vi "ReadChanValue.vi"(8 "error in (no error)":errorcluster, 10 "nScale":i32, 11 "nWhichChan":i32) -> (0 "error out":errorcluster, 1 "*pnChanSpanOffset":i32, 2 "*pnChanZeroOffset":i32, 3 "Return Code":i32, 5 "*pnChanValue":i32)   [LabVIEW 2015]
doc: "Call this to initiate a connection with the UUT. \nDetail: \nint ConnectToOthello (aMEScope_ReadChanVal\nDescription:\nThis function will read an analog channel ADC offset. Calibration values are also returned to properly calculate the final result.\nDetail:\nint MEScope_ReadChanVal (\nint nWhichChan, \nint nScale, \nint *pnChanValue, \nint *pnChanZeroOffset,\nint *pnChanSpanOffset\n);\nParameters:\nint nWhichChan - which channel to use (CHANNEL_1 or CHANNEL_2)\n\nint nScale - which scale to use (CHANNEL_SCALE_1V to CHANNEL_SCALE_400V)\n\nint *pnChanValue - pointer to an integer, filled with the ADC count value for the channel, scale and input requested.\n\nint * pnChanZeroOffset - pointer to an integer, filled with the zero offset calibration value for the requested channel, scale and input. It can be NULL if the data isn't required.\n\nint * pnChanSpanOffset - pointer to an integer, filled with the span offset calibration value for the requested channel, scale and input. It can be NULL if the data isn't required.\n\nReturn Values:\nThis function returns a 0 if the function completed successfully. A non-zero return code will indicate error. \nRemarks:\nChannel definitions:\n#define CHANNEL_1 0\n#define CHANNEL_2 1\n\nScale definitions:\n#define CHANNEL_SCALE_1V 0\n#define CHANNEL_SCALE_2V 1\n#define CHANNEL_SCALE_5V 2\n#define CHANNEL_SCALE_10V 3\n#define CHANNEL_SCALE_20V 4\n#define CHANNEL_SCALE_50V 5\n#define CHANNEL_SCALE_100V 6\n#define CHANNEL_SCALE_200V 7\n#define CHANNEL_SCALE_400V 8\n\nSee Appendix 4 for details on converting ADC reading into a measurement.\nSerial Command packet: \nn/a\n\nint nPort\n);\n \nParameters:\nint nPort - Port used by USB serial device\nReturn Values:\nA returned value of 0 indicates success. A non-zero return code will indicate error.\nRemarks:"
uses:
  ScannerDiagDLL.dll
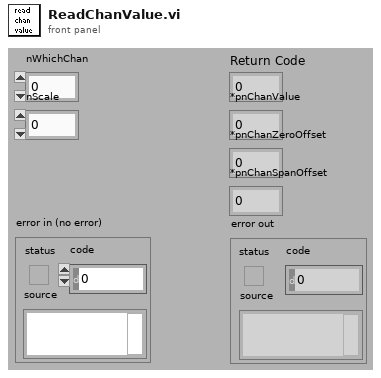
[diagram p1: front panel]
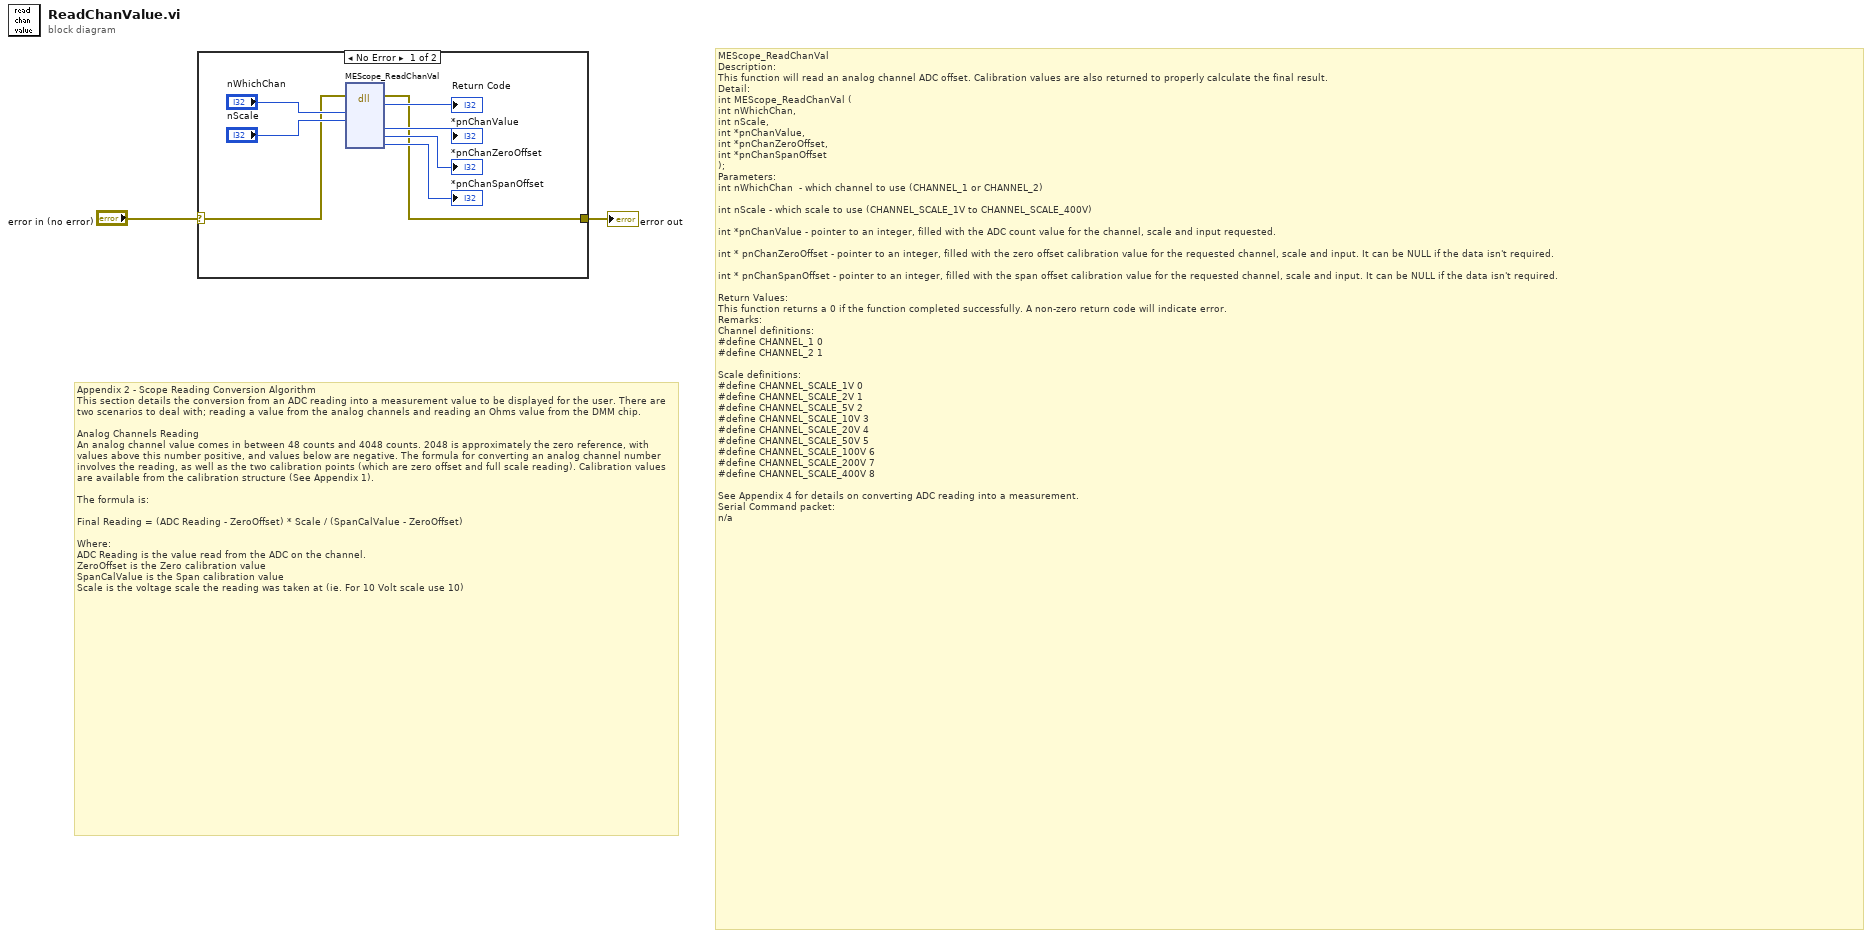
[diagram p0: block diagram]
diagram:
  # "Appendix 2 - Scope Reading Conversion Algorithm\nThis section details the conversion from an ADC reading into a measurement value to be displayed for the user. There are two scenarios to deal with; reading a value from the analog channels and reading an Ohms value from the DMM chip.\n\nAnalog Channels Reading\nAn analog channel value comes in between 48 counts and 4048 counts. 2048 is approximately the zero reference, with values above this number positive, and values below are negative. The formula for converting an analog channel number involves the reading, as well as the two calibration points (which are zero offset and full scale reading). Calibration values are available from the calibration structure (See Appendix 1). \n\nThe formula is:\n\nFinal Reading = (ADC Reading - ZeroOffset) * Scale / (SpanCalValue - ZeroOffset)\n\nWhere:\nADC Reading is the value read from the ADC on the channel.\nZeroOffset is the Zero calibration value\nSpanCalValue is the Span calibration value\nScale is the voltage scale the reading was taken at (ie. For 10 Volt scale use 10)"
  # "MEScope_ReadChanVal\nDescription:\nThis function will read an analog channel ADC offset. Calibration values are also returned to properly calculate the final result.\nDetail:\nint MEScope_ReadChanVal (\nint nWhichChan, \nint nScale, \nint *pnChanValue, \nint *pnChanZeroOffset,\nint *pnChanSpanOffset\n);\nParameters:\nint nWhichChan  - which channel to use (CHANNEL_1 or CHANNEL_2)\n\nint nScale - which scale to use (CHANNEL_SCALE_1V to CHANNEL_SCALE_400V)\n\nint *pnChanValue - pointer to an integer, filled with the ADC count value for the channel, scale and input requested.\n\nint * pnChanZeroOffset - pointer to an integer, filled with the zero offset calibration value for the requested channel, scale and input. It can be NULL if the data isn't required.\n\nint * pnChanSpanOffset - pointer to an integer, filled with the span offset calibration value for the requested channel, scale and input. It can be NULL if the data isn't required.\n\nReturn Values:\nThis function returns a 0 if the function completed successfully. A non-zero return code will indicate error. \nRemarks:\nChannel definitions:\n#define CHANNEL_1\t0\n#define CHANNEL_2\t1\n\nScale definitions:\n#define CHANNEL_SCALE_1V\t0\n#define CHANNEL_SCALE_2V\t1\n#define CHANNEL_SCALE_5V\t2\n#define CHANNEL_SCALE_10V\t3\n#define CHANNEL_SCALE_20V\t4\n#define CHANNEL_SCALE_50V\t5\n#define CHANNEL_SCALE_100V\t6\n#define CHANNEL_SCALE_200V\t7\n#define CHANNEL_SCALE_400V\t8\n\nSee Appendix 4 for details on converting ADC reading into a measurement.\nSerial Command packet: \nn/a"
  n1 = case shown="No Error" "error in (no error)" {
    selector: "error in (no error)" -> [w4 w11]
    tunnel: [w3 w11] -> w1
    frame No Error {
      n2 = dll-call lib="C:/ModisEdge/Scope/Test Sequence/Code Modules/DLL/ScannerDiagDLL.dll" fn="MEScope_ReadChanVal" ("TripoliDLL.dll:Test_WirelessLANPort")(error in=w4, "nWhichChan"="nWhichChan", "nScale"="nScale") -> (error out=w3:errorcluster, "return type"=→"Return Code":i32, "pnChanValue"=→"*pnChanValue":i32, "pnChanZeroOffset"=→"*pnChanZeroOffset":i32, "pnChanSpanOffset"=→"*pnChanSpanOffset":i32)  [unwired: 7 in, 1 out]
    }
    frame Error {
    }
  }
  "error out" <- w1
